vi "Load_All_Transconductance.vi"() -> ()   [LabVIEW 2016]
panel:
  in  "flatten?":bool
  in  "Numeric 2":i32
  in  "New Files to Process":string="P:\\expt\\PPMS data\\SA02836H.20160926\\03-LockinVsgB_fine"
  out "Array 4":dbl[](array[numeric])
  out "Intensity Graph 17":dbl[][](graph)
  out "B fields":dbl[][](array[numeric])
  out "Numeric":i32=37
  out "Array":i32[][](array[numeric])=[[122, 457], [122, 457], [122, 457], [122, 457], [120, 457], [121, 457], [120, 457], [121, 457], [120, 457], [121, 457], [121, 457], [121, 457], [121, 457], [121, 457], [120, 457], [121, 457], [120, 457], [121, 457], [121, 457], [121, 457], [121, 457], [121, 457], [120, 457], [121, 457], [121, 457], [121, 457], [121, 457], [121, 457], [121, 457], [121, 457], [121, 457], [121, 457], [121, 457], [121, 457], [120, 457], [121, 457], [121, 457], [121, 457]]
  in  "read data from file?":bool=TRUE
  out "angle":dbl=44.0
  out "Vsg":dbl=63.54485776805251
  out "B field":dbl=9.0
  out "Intensity Graph 12":dbl[][][](array[numeric])
  out "Intensity Graph 16":dbl[][](graph)
  out "Intensity Graph 15":dbl[][](graph)
  out "Intensity Graph 14":dbl[][](graph)
  in  "angle index":i32=22
  # "P:\\expt\\Leiden MNK\\SA02836H.20170110\\9\\9-sweep B, angle,, Vsg Lockin-0\nP:\\expt\\Leiden MNK\\SA02836H.20170110\\9\\9-sweep B, angle,, Vsg Lockin-1\nP:\\expt\\Leiden MNK\\SA02836H.20170110\\9\\9-sweep B, angle,, Vsg Lockin-2\nP:\\expt\\Leiden MNK\\SA02836H.20170110\\9\\9-sweep B, angle,, Vsg Lockin-3\nP:\\expt\\Leiden MNK\\SA02836H.20170110\\9\\9-sweep B, angle,, Vsg Lockin-4\nP:\\expt\\Leiden MNK\\SA02836H.20170110\\9\\9-sweep B, angle,, Vsg Lockin-5\nP:\\expt\\Leiden MNK\\SA02836H.20170110\\9A\\9A-sweep B, angle, Vsg Lockin-0\nP:\\expt\\Leiden MNK\\SA02836H.20170110\\9A\\9A-sweep B, angle, Vsg Lockin-1\nP:\\expt\\Leiden MNK\\SA02836H.20170110\\9A\\9A-sweep B, angle, Vsg Lockin-2\nP:\\expt\\Leiden MNK\\SA02836H.20170110\\9A\\9A-sweep B, angle, Vsg Lockin-3\nP:\\expt\\Leiden MNK\\SA02836H.20170110\\9A\\9A-sweep B, angle, Vsg Lockin-4\nP:\\expt\\Leiden MNK\\SA02836H.20170110\\9A\\9A-sweep B, angle, Vsg Lockin-5\nP:\\expt\\Leiden MNK\\SA02836H.20170110\\9A\\9A-sweep B, angle, Vsg Lockin-6\nP:\\expt\\Leiden MNK\\SA02836H.20170110\\9A\\9A-sweep B, angle, Vsg Lockin-7\nP:\\expt\\Leiden MNK\\SA02836H.20170110\\9A\\9A-sweep B, angle, Vsg Lockin-8\nP:\\expt\\Leiden MNK\\SA02836H.20170110\\9A\\9A-sweep B, angle, Vsg Lockin-9\nP:\\expt\\Leiden MNK\\SA02836H.20170110\\9B\\9B-sweep B, angle, Vsg Lockin-0\nP:\\expt\\Leiden MNK\\SA02836H.20170110\\9B\\9B-sweep B, angle, Vsg Lockin-1\nP:\\expt\\Leiden MNK\\SA02836H.20170110\\9C\\9C-sweep B, angle, Vsg Lockin-0\nP:\\expt\\Leiden MNK\\SA02836H.20170110\\9C\\9C-sweep B, angle, Vsg Lockin-1\nP:\\expt\\Leiden MNK\\SA02836H.20170110\\9C\\9C-sweep B, angle, Vsg Lockin-2\nP:\\expt\\Leiden MNK\\SA02836H.20170110\\9C\\9C-sweep B, angle, Vsg Lockin-3\nP:\\expt\\Leiden MNK\\SA02836H.20170110\\9C\\9C-sweep B, angle, Vsg Lockin-4\nP:\\expt\\Leiden MNK\\SA02836H.20170110\\9C\\9C-sweep B, angle, Vsg Lockin-5\nP:\\expt\\Leiden MNK\\SA02836H.20170110\\9C\\9C-sweep B, angle, Vsg Lockin-6\nP:\\expt\\Leiden MNK\\SA02836H.20170110\\9C\\9C-sweep B, angle, Vsg Lockin-7\nP:\\expt\\Leiden MNK\\SA02836H.20170110\\9D\\9D-sweep B, angle, Vsg Lockin-0\nP:\\expt\\Leiden MNK\\SA02836H.20170110\\9D\\9D-sweep B, angle, Vsg Lockin-1\nP:\\expt\\Leiden MNK\\SA02836H.20170110\\9D\\9D-sweep B, angle, Vsg Lockin-2\nP:\\expt\\Leiden MNK\\SA02836H.20170110\\9D\\9D-sweep B, angle, Vsg Lockin-3\nP:\\expt\\Leiden MNK\\SA02836H.20170110\\9D\\9D-sweep B, angle, Vsg Lockin-4\nP:\\expt\\Leiden MNK\\SA02836H.20170110\\9D\\9D-sweep B, angle, Vsg Lockin-5\nP:\\expt\\Leiden MNK\\SA02836H.20170110\\9D\\9D-sweep B, angle, Vsg Lockin-6\nP:\\expt\\Leiden MNK\\SA02836H.20170110\\9D\\9D-sweep B, angle, Vsg Lockin-7\nP:\\expt\\Leiden MNK\\SA02836H.20170110\\9D\\9D-sweep B, angle, Vsg Lockin-8\nP:\\expt\\Leiden MNK\\SA02836H.20170110\\9D\\9D-sweep B, angle, Vsg Lockin-9\nP:\\expt\\Leiden MNK\\SA02836H.20170110\\9D\\x9D-sweep B, angle, Vsg Lockin-10\nP:\\expt\\Leiden MNK\\SA02836H.20170110\\9D\\x9D-sweep B, angle, Vsg Lockin-11\nP:\\expt\\Leiden MNK\\SA02836H.20170110\\9D\\x9D-sweep B, angle, Vsg Lockin-12\nP:\\expt\\Leiden MNK\\SA02836H.20170110\\9D\\x9D-sweep B, angle, Vsg Lockin-13\nP:\\expt\\Leiden MNK\\SA02836H.20170110\\9E\\9E-sweep B, angle, Vsg Lockin-0\nP:\\expt\\Leiden MNK\\SA02836H.20170110\\9E\\9E-sweep B, angle, Vsg Lockin-1\nP:\\expt\\Leiden MNK\\SA02836H.20170110\\9E\\9E-sweep B, angle, Vsg Lockin-2\nP:\\expt\\Leiden MNK\\SA02836H.20170110\\9E\\9E-sweep B, angle, Vsg Lockin-3\nP:\\expt\\Leiden MNK\\SA02836H.20170110\\9E\\9E-sweep B, angle, Vsg Lockin-4"
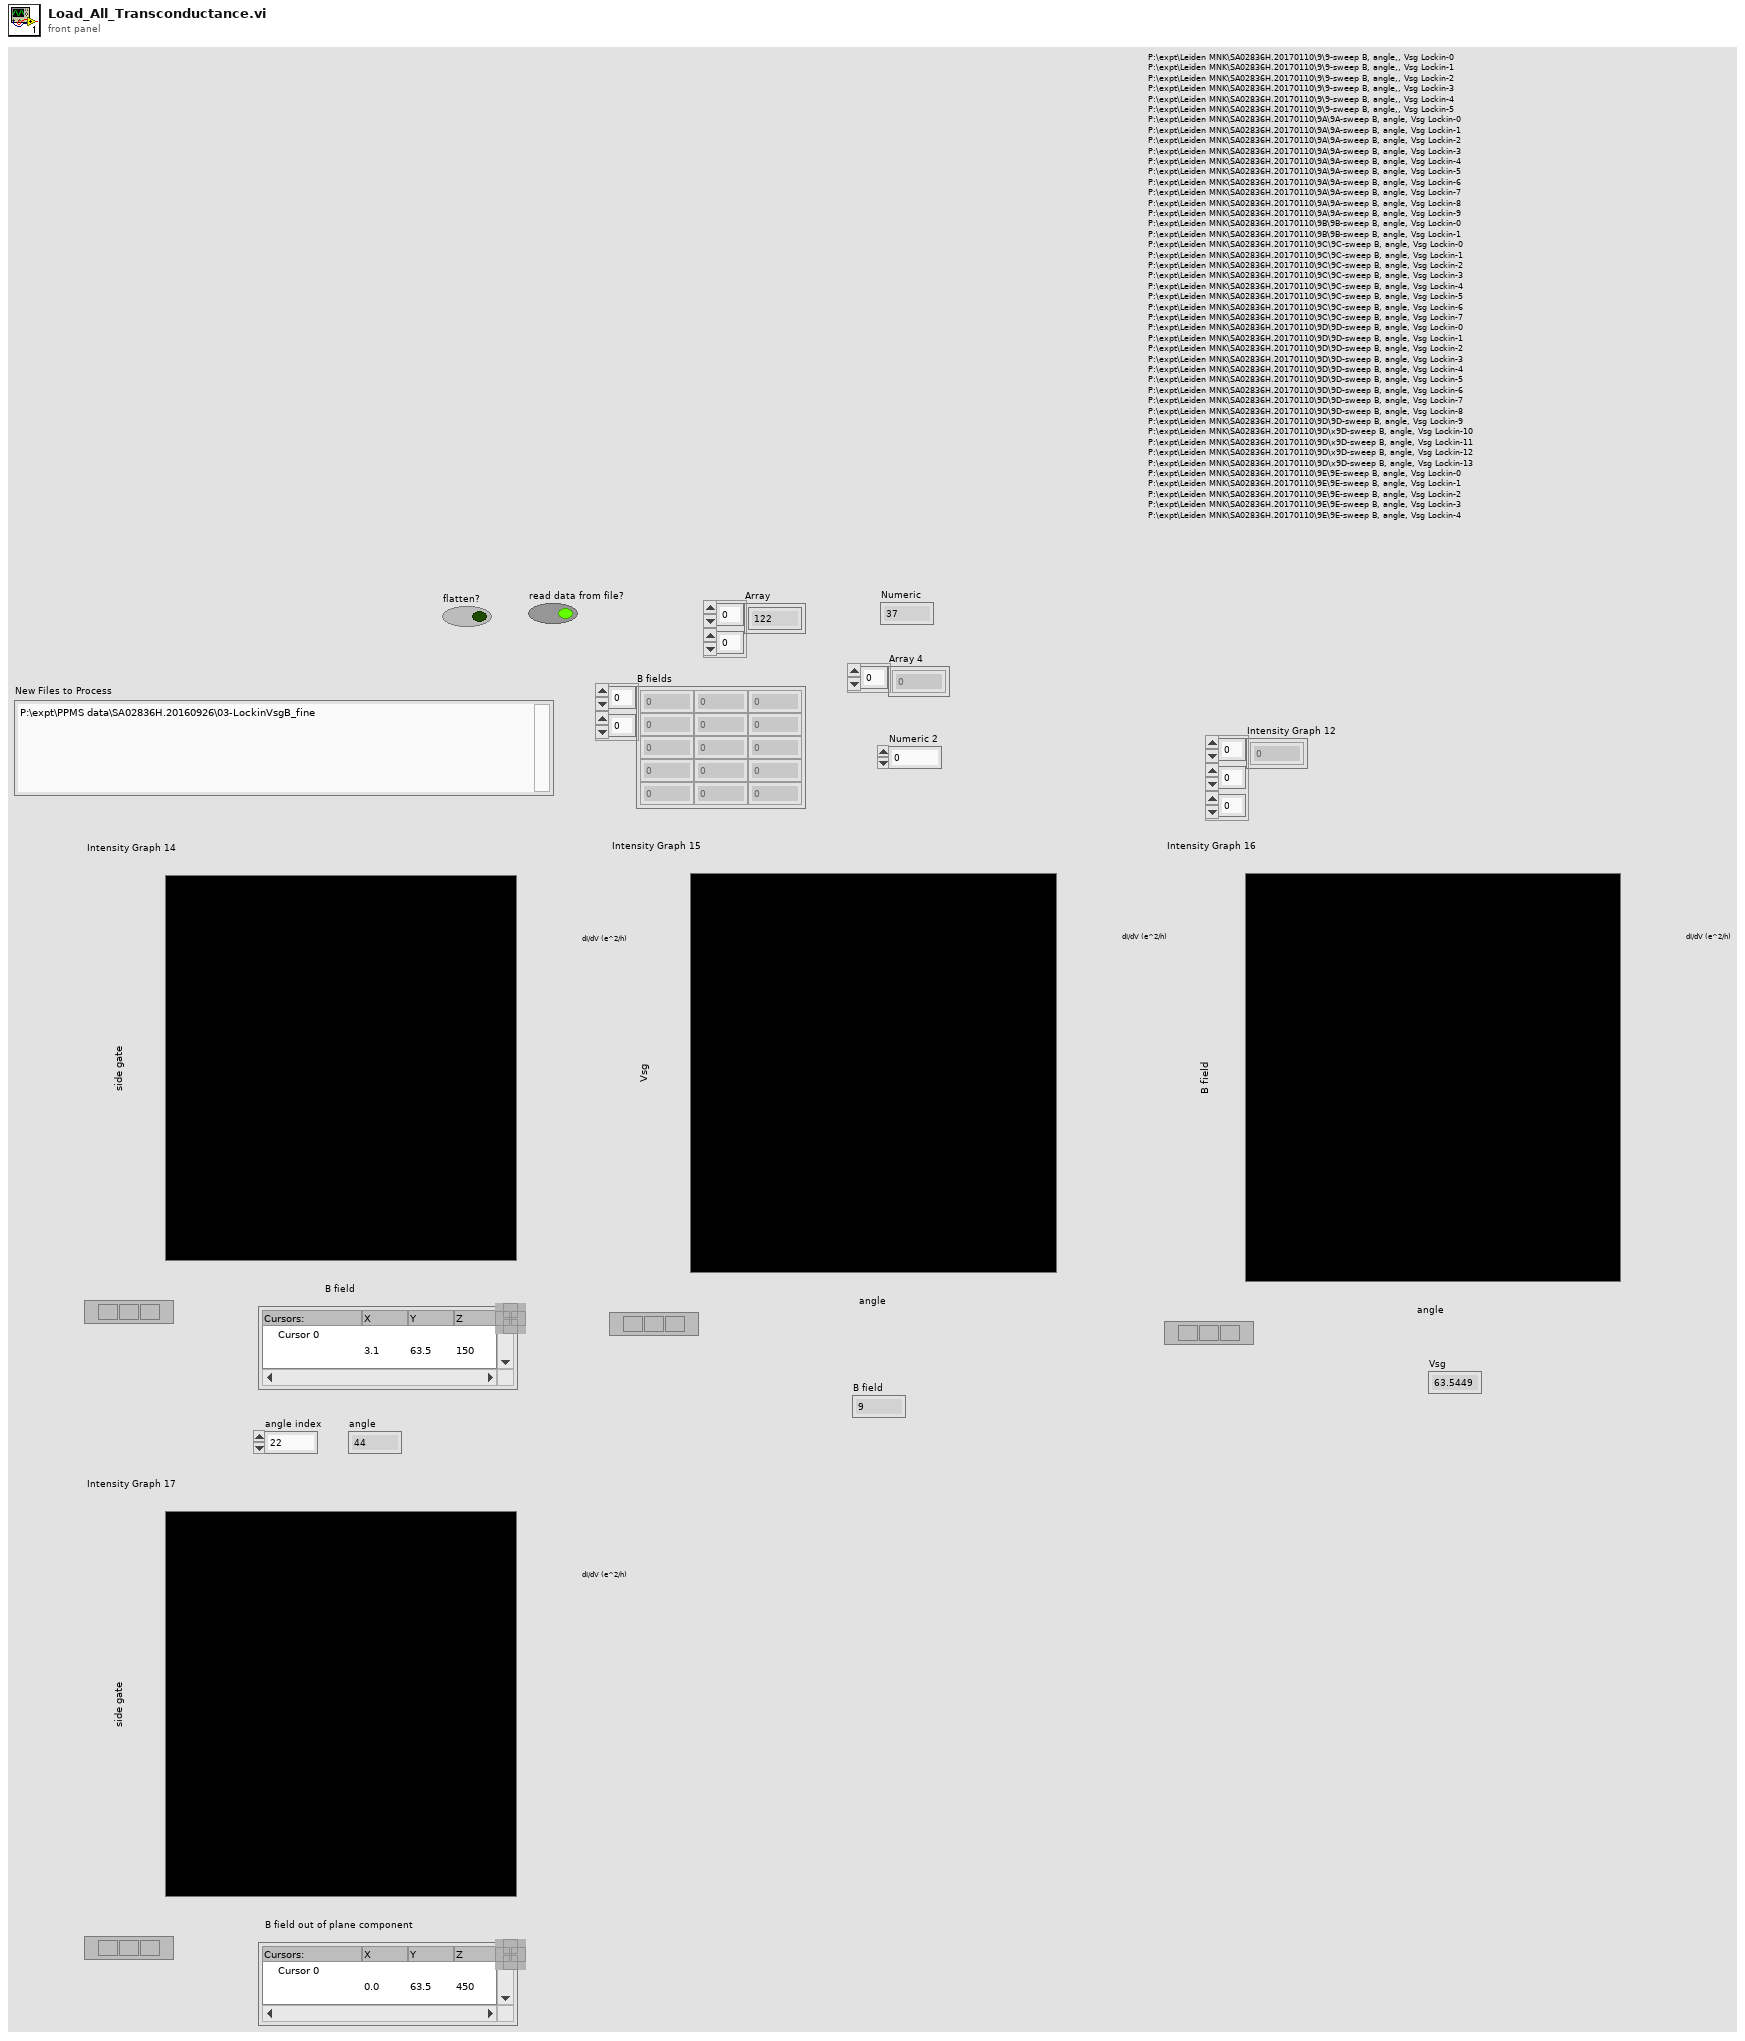
[diagram p1: front panel]
types:
  T1 = cluster{"N1":dbl, "N2":dbl, "N3":dbl, "N4":dbl}[]
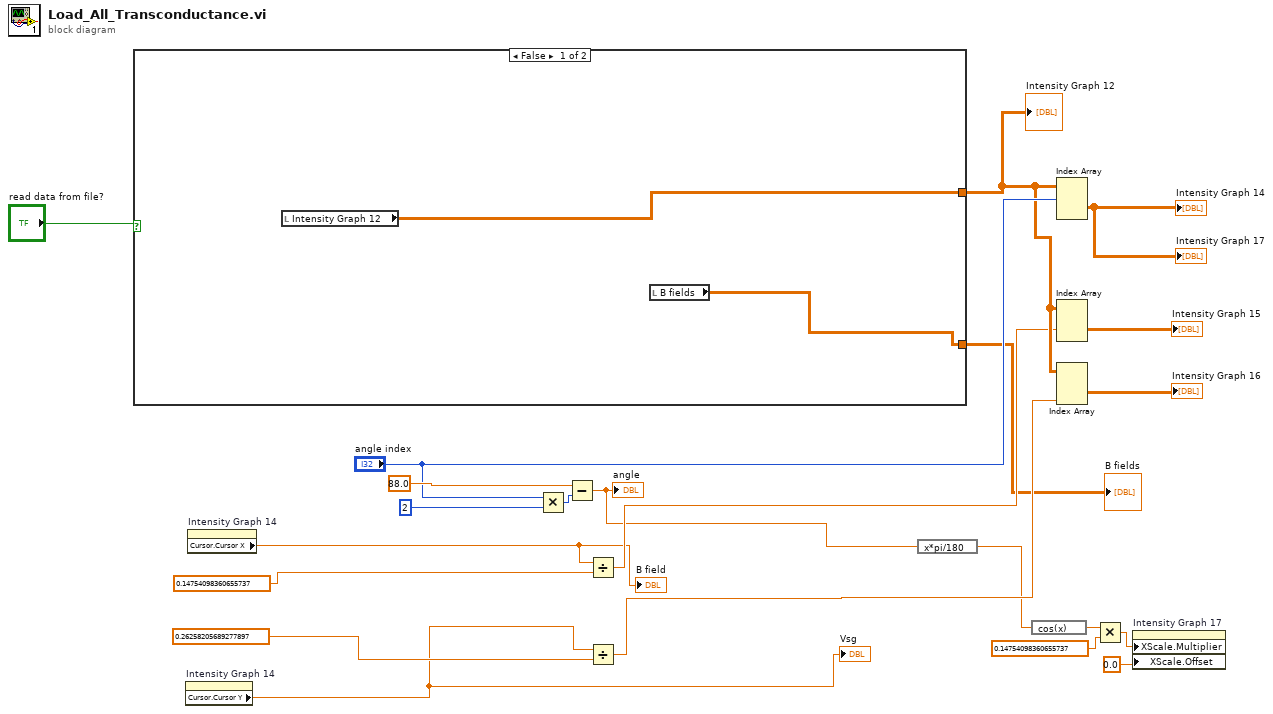
[diagram p0: block diagram]
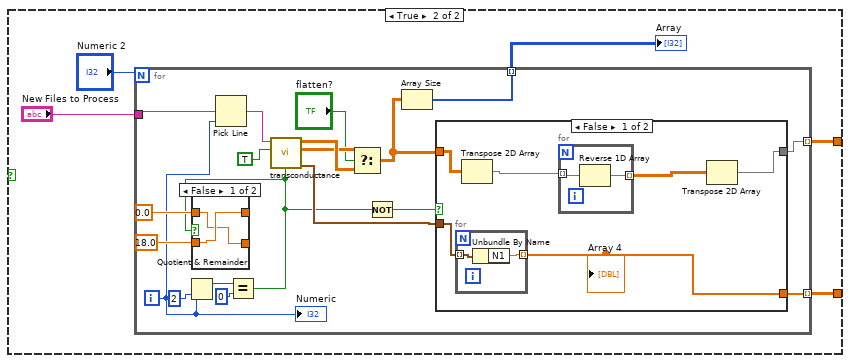
[diagram p2: hidden frame]
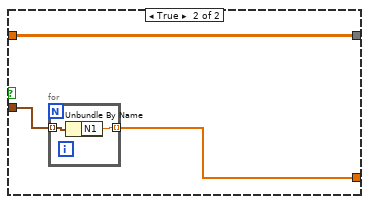
[diagram p4: hidden frame]
diagram:
  n1 = case shown="False" "read data from file?" {
    tunnel: [w24 w29] -> w15
    tunnel: [w23 w27] -> w8
    frame False {
      n2 = local read "Intensity Graph 12"() -> (w24:dbl[][][])
      n3 = local read "B fields"() -> (w23:dbl[][])
    }
    frame True {
      n4 = for {
        N: "Numeric 2" -> [_]
        tunnel: [w48] -> w29 mode=indexing
        tunnel: [w47] -> w28 mode=indexing
        tunnel: [w45] -> w27 mode=indexing
        tunnel: "New Files to Process" -> [w39]
        i -> [w38]
        n5 = Quotient & Remainder(x=w38, y=2) -> (x-y*floor(x/y)=w41:i32)  [unwired: 1 out]
        n6 = Pick Line(multi-line string=w39, line index=w38) -> (output string=w37:string)  [unwired: 1 in]
        n7 = Equal?(x=w41, y=0) -> (x = y?=w30:bool)
        n8 = case shown="False" w30 {
          tunnel: 0.0 ("B min") -> [w49 w52]
          tunnel: [w50 w52] -> _
          tunnel: 18.0 ("B max") -> [w50 w51]
          tunnel: [w49 w51] -> _
          frame False {
          }
          frame True {
          }
        }
        n9 = call "transconductance.vi"("reverse flattening array?"=w30, "load data from file?"=TRUE, "New Files to Process"=w37) -> ("N Array"=w46:T1, "adjusted trans"=w33:dbl[][], "Intensity Graph 12"=w34:dbl[][])  [unwired: 3 in, 3 out]
        n10 = Select(t=w33, s="flatten?", f=w34) -> (s? t:f=w35:dbl[][])
        n11 = Not(x=w30) -> (.not. x?=w31:bool)
        n12 = Array Size(array=w35) -> (size(s)=w47:i32[])
        n13 = case shown="False" w31 {
          tunnel: w35 -> [w58 w65]
          tunnel: [w55 w65] -> w48
          tunnel: w46 -> [w54 w64]
          tunnel: [w53 w63] -> w45
          frame False {
            n14 = for {
              tunnel: w54 -> [w60] mode=indexing
              tunnel: [w59] -> w53 mode=indexing
              n15 = Unbundle By Name(w60) -> ("N1"=w59:dbl)
            }
            "Array 4" <- w53
            n16 = Transpose 2D Array(2D array=w58) -> (transposed array=w57:dbl[][])
            n17 = for {
              tunnel: w57 -> [w62] mode=indexing
              tunnel: [w61] -> w56 mode=indexing
              n18 = Reverse 1D Array(array=w62) -> (reversed array=w61:dbl[])
            }
            n19 = Transpose 2D Array(2D array=w56) -> (transposed array=w55:dbl[][])
          }
          frame True {
            n20 = for {
              tunnel: w64 -> [w67] mode=indexing
              tunnel: [w66] -> w63 mode=indexing
              n21 = Unbundle By Name(w67) -> ("N1"=w66:dbl)
            }
          }
        }
        "Numeric" <- w38
      }
      "Array" <- w28
    }
  }
  "Intensity Graph 12" <- w15
  "B fields" <- w8
  n22 = property on="Intensity Graph 14" class="IntGraph (strict)"() -> ("Cursor.Cursor Y"=w10:dbl)  [unwired: 2 in, 2 out]
  "Vsg" <- w10
  n23 = property on="Intensity Graph 14" class="IntGraph (strict)"() -> ("Cursor.Cursor X"=w12:dbl)  [unwired: 2 in, 2 out]
  "B field" <- w12
  n24 = Multiply(x="angle index", y=2) -> (x*y=w18:i32)
  n25 = Subtract(x=88.0, y=w18) -> (x-y=w2:dbl)
  "angle" <- w2
  n26 = Divide(x=w12, y=0.14754098360655737) -> (x/y=w13:dbl)
  n27 = Divide(x=w10, y=0.26258205689277897) -> (x/y=w11:dbl)
  n28 = expression code="x*pi/180"(w2) -> (w1:dbl)
  n29 = expression code="cos(x)"(w1) -> (w4:dbl)
  n30 = Index Array(array=w15, index (dim 0)="angle index") -> (element=→"Intensity Graph 14" →"Intensity Graph 17":dbl[][])  [unwired: 2 in]
  n31 = Index Array(array=w15, index (dim 1)=w13) -> (element=→"Intensity Graph 15":dbl[][])  [unwired: 2 in]
  n32 = Index Array(array=w15, index (dim 2)=w11) -> (element=→"Intensity Graph 16":dbl[][])  [unwired: 2 in]
  n33 = Multiply(x=w4, y=0.14754098360655737) -> (x*y=w3:dbl)
  n34 = property on="Intensity Graph 17" class="IntGraph (strict)"("XScale.Multiplier"=w3, "XScale.Offset"=0.0) -> ()  [unwired: 2 in, 2 out]
